vi "Func-패킷 프로토콜-패킷 조립.vi"(4 "메시지 데이터":string, 5 "ID":u8 format="%02d") -> (2 "패킷 데이터 (Hex)":string)   [LabVIEW 2015]
panel:
  out "패킷 전체 길이":i32
  # "* 패킷 프로토콜 - 프레임 데이터 전송"
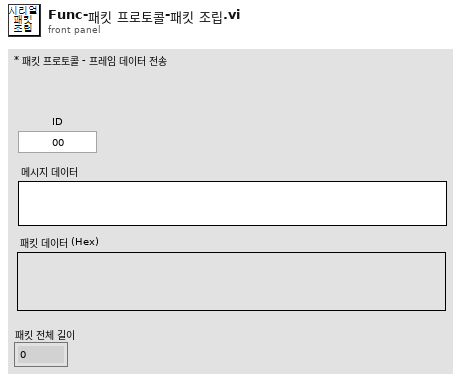
[diagram p1: front panel]
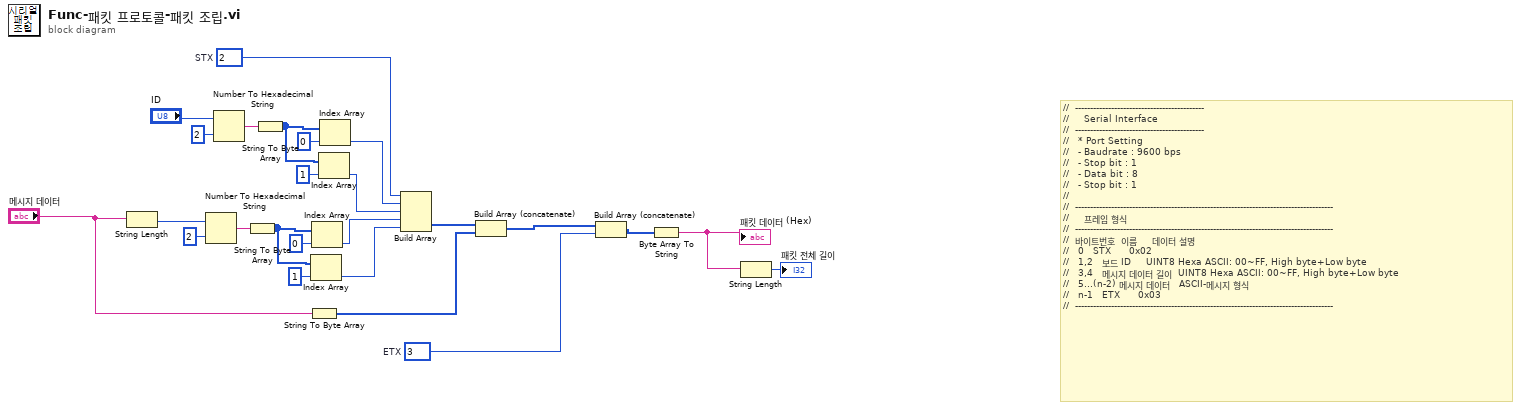
[diagram p0: block diagram]
diagram:
  w1 = u8 3  # ETX
  w15 = u8 2  # STX
  # "//\t\t-------------------------------------------\n//\t\t\t\t\tSerial Interface\n//\t\t-------------------------------------------\n//\t\t\t* Port Setting\n//\t\t\t- Baudrate : 9600 bps\n//\t\t\t- Stop bit : 1\n//\t\t\t- Data bit : 8 \n//\t\t\t- Stop bit : 1\t\n//\n//\t\t--------------------------------------------------------------------------------------\n//\t\t\t\t\t프레임 형식\n//\t\t--------------------------------------------------------------------------------------\n//\t\t바이트번호\t\t이름\t\t\t\t\t데이터 설명\n//\t\t\t0\t\t\tSTX \t\t\t\t\t0x02\n//\t\t\t1,2\t\t\t보드 ID \t\t\t\tUINT8 Hexa ASCII: 00~FF, High byte+Low byte\n//\t\t\t3,4\t\t\t메시지 데이터 길이\t\tUINT8 Hexa ASCII: 00~FF, High byte+Low byte\n//\t\t\t5...(n-2)\t메시지 데이터\t\t\tASCII-메시지 형식\n//\t\t\tn-1\t\t\tETX \t\t\t\t\t0x03\n//\t\t--------------------------------------------------------------------------------------"
  n1 = String Length(string="메시지 데이터") -> (length=w4:i32)
  n2 = Number To Hexadecimal String(1:i16 2 ("폭(-)"), 2:w4) -> (0:w6:string)
  n3 = Number To Hexadecimal String(1:i16 2 ("폭(-)"), 2:"ID") -> (0:w16:string)
  n4 = String To Byte Array(string=w6) -> (unsigned byte array=w9:u8[])
  n5 = String To Byte Array(string=w16) -> (unsigned byte array=w12:u8[])
  n6 = String To Byte Array(string="메시지 데이터") -> (unsigned byte array=w24:u8[])
  n7 = Index Array(array=w9, index=1 ("인덱스")) -> (element=w2:u8)
  n8 = Index Array(array=w9, index=0 ("인덱스")) -> (element=w3:u8)
  n9 = Index Array(array=w12, index=1 ("인덱스")) -> (element=w10:u8)
  n10 = Index Array(array=w12, index=0 ("인덱스")) -> (element=w11:u8)
  n11 = Build Array(w15, w11, w10, w3, w2) -> (w22:u8[])
  n12 = Build Array (concatenate)(w22, w24) -> (w23:u8[])
  n13 = Build Array (concatenate)(w23, w1) -> (w25:u8[])
  n14 = Byte Array To String(unsigned byte array=w25) -> (string=w20:string)
  "패킷 데이터 (Hex)" <- w20
  n15 = String Length(string=w20) -> (length=→"패킷 전체 길이":i32)
